vi "Preset PASS HOLD time.vi"(8 "error in (no error)":errorcluster, 10 "Step Time":dbl=0.2 min=0.2 max=99.9 step=0.1 format="%.1f", 11 "VISA resource in":refnum<visa-resource-name>) -> (0 "error out":errorcluster, 3 "VISA resource out":refnum<visa-resource-name>)   [LabVIEW 2025, in "Chroma 19572.lvlib"]
doc: "This VI writes to the instrument the PASS HOLD time."
uses:
  <instrlib>/Chroma 19572/Chroma 19572.lvlib
panel:
  # "[sec]"
  # "PreSet PASS HOLD Time"
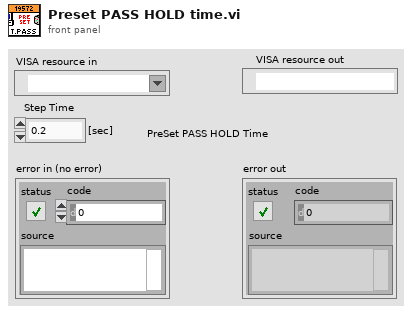
[diagram p1: front panel]
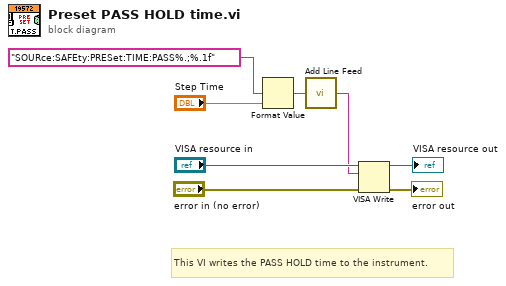
[diagram p0: block diagram]
diagram:
  # "This VI writes the PASS HOLD time to the instrument."
  n1 = Format Value(format string="SOURce:SAFEty:PRESet:TIME:PASS%.;%.1f", value (0)="Step Time") -> (output string=w2:string)  [unwired: 1 in]
  n2 = call <instrlib>:"Add Line Feed.vi"("Command string"=w2) -> ("Concatenated string"=w1:string)  [unwired: 4 in]
  n3 = VISA Write(VISA resource name="VISA resource in", write buffer=w1, error in (no error)="error in (no error)") -> (VISA resource name out=→"VISA resource out":refnum<visa-resource-name>, error out=→"error out":errorcluster)  [unwired: 1 out]
